vi "test Conversion from Name to Symbol.vi"(8 "error in":errorcluster, 11 "TestCase in":refnum<class "Refresh.lvclass">) -> (0 "error out":errorcluster, 3 "TestCase out":refnum<class "Refresh.lvclass">)   [LabVIEW 2020, in "Refresh.lvclass"]
uses:
  Refresh.lvclass
  <vilib>/addons/_JKI Toolkits/VI Tester/TestCase.llb/TestCase.lvclass
  System Explorer/Implementation/System Explorer/Refresh/Refresh.lvlib
  Scripting/Constants.vi
  Scripting/AIM MIL-STD-1553 Scripting.lvlib
  System Explorer/Implementation/System Explorer/Refresh/Symbols.ctl
  C:/Program Files (x86)/National Instruments/LabVIEW 2020/vi.lib/addons/_JKI Toolkits/VI Tester/TestCase.llb/TestCase.lvclass
  C:/Users/nitest/Desktop/clonetemp/Custom Device Support/Tests/Unit/Refresh/Refresh.lvclass
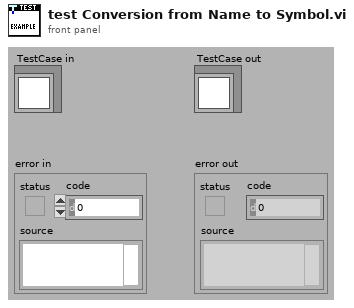
[diagram p1: front panel]
types:
  T1 = typedef "AIM MIL-STD-1553 System Explorer.lvlib/Implementation.lvlib/Refresh.lvlib/Symbols.ctl" = enum16{"Blank", "MIL-STD-1553", "Port", "Remote Terminal", "Subaddress", "Bus Controller", "Acyclic Frame", "Mode Code", "Message", "Parameter", "Item"}
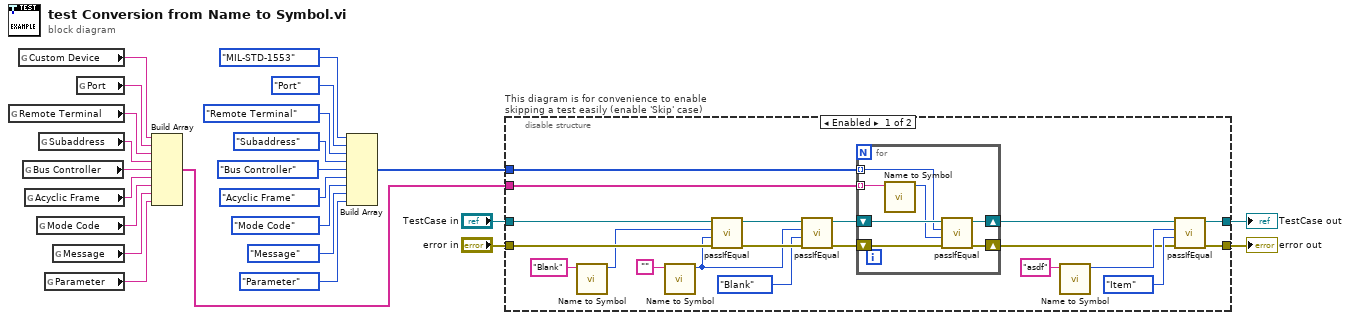
[diagram p0: block diagram]
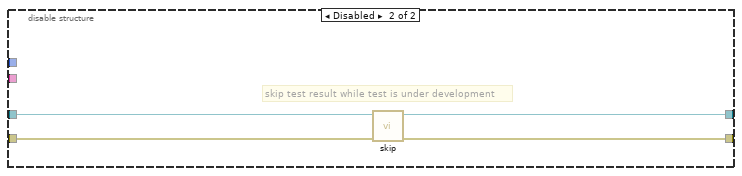
[diagram p2: hidden frame]
diagram:
  n1 = global read "Constants.vi" "Remote Terminal"() -> (w4:string)
  n2 = global read "Constants.vi" "Custom Device"() -> (w2:string)
  n3 = global read "Constants.vi" "Bus Controller"() -> (w6:string)
  n4 = global read "Constants.vi" "Acyclic Frame"() -> (w7:string)
  n5 = global read "Constants.vi" "Mode Code"() -> (w8:string)
  n6 = global read "Constants.vi" "Subaddress"() -> (w5:string)
  n7 = global read "Constants.vi" "Parameter"() -> (w10:string)
  n8 = global read "Constants.vi" "Message"() -> (w9:string)
  n9 = global read "Constants.vi" "Port"() -> (w3:string)
  n10 = Build Array(w2, w3, w4, w5, w6, w7, w8, w9, w10) -> (w1:string[])
  n11 = Build Array(Symbols."MIL-STD-1553" ("item symbol"), Symbols."Port" ("item symbol"), Symbols."Remote Terminal" ("item symbol"), Symbols."Subaddress" ("item symbol"), Symbols."Bus Controller" ("item symbol"), Symbols."Acyclic Frame" ("item symbol"), Symbols."Mode Code" ("item symbol"), Symbols."Message" ("item symbol"), Symbols."Parameter" ("item symbol")) -> (w19:T1[])
  n12 = disable-structure "This diagram is for convenience to enable skipping a test easily (enable 'Skip' case)" shown="Enabled" {
    disable-tunnel: "TestCase in" -> [w44 w55]
    disable-tunnel: [w26 w53] -> w21
    disable-tunnel: [w25 w54] -> w23
    disable-tunnel: "error in" -> [w43 w52]
    disable-tunnel: w19 -> [w33 _]
    disable-tunnel: w1 -> [w32 _]
    frame Enabled {
      n13 = call "Name to Symbol.vi"("item name"="Blank") -> ("item symbol"=w40:T1)  [unwired: 10 in]
      n14 = call "Name to Symbol.vi"("item name"="") -> ("item symbol"=w36:T1)  [unwired: 10 in]
      n15 = call-dynamic "passIfEqual.vi"("error in (no error)"=w43, "y"=w36, "x"=w40, "TestCase in"=w44) -> ("error out"=w38:errorcluster, "TestCase out"=w39:refnum<class "Refresh.lvclass">)  [unwired: 6 in]
      n16 = call-dynamic "passIfEqual.vi"("error in (no error)"=w38, "y"=Symbols."Blank" ("item symbol"), "x"=w36, "TestCase in"=w39) -> ("error out"=w34:errorcluster, "TestCase out"=w35:refnum<class "Refresh.lvclass">)  [unwired: 6 in]
      n17 = for {
        shift-right: [w49] -> w28
        shift-left: w35 -> [w51]
        shift-right: [w48] -> w27
        shift-left: w34 -> [w50]
        tunnel: w32 -> [w47] mode=indexing
        tunnel: w33 -> [w45] mode=indexing
        n18 = call "Name to Symbol.vi"("item name"=w47) -> ("item symbol"=w46:T1)  [unwired: 10 in]
        n19 = call-dynamic "passIfEqual.vi"("error in (no error)"=w50, "y"=w46, "x"=w45, "TestCase in"=w51) -> ("error out"=w48:errorcluster, "TestCase out"=w49:refnum<class "Refresh.lvclass">)  [unwired: 6 in]
      }
      n20 = call "Name to Symbol.vi"("item name"="asdf") -> ("item symbol"=w30:T1)  [unwired: 10 in]
      n21 = call-dynamic "passIfEqual.vi"("error in (no error)"=w27, "y"=Symbols."Item" ("item symbol"), "x"=w30, "TestCase in"=w28) -> ("error out"=w25:errorcluster, "TestCase out"=w26:refnum<class "Refresh.lvclass">)  [unwired: 6 in]
    }
    frame Disabled {
      # "skip test result while test is under development"
      n22 = call <vilib>:"skip.vi"("error in (no error)"=w52, "TestCase in"=w55) -> ("error out"=w54:errorcluster, "TestCase out"=w53:refnum<class "Refresh.lvclass">)  [unwired: 8 in]
    }
  }
  "error out" <- w23
  "TestCase out" <- w21
